vi "Start Async.vi"(8 "error in (no error)":errorcluster, 11 "OOP Server in":refnum<class "Template Server.lvclass">) -> (0 "error out":errorcluster, 3 "OOP Server out":refnum<class "Template Server.lvclass">)   [LabVIEW 2019, in "Template Server.lvlib" / "Template Server.lvclass"]
uses:
  Template Server.lvclass
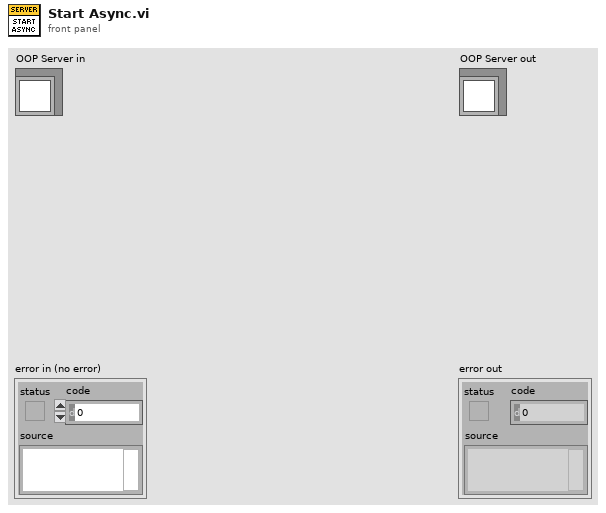
[diagram p1: front panel]
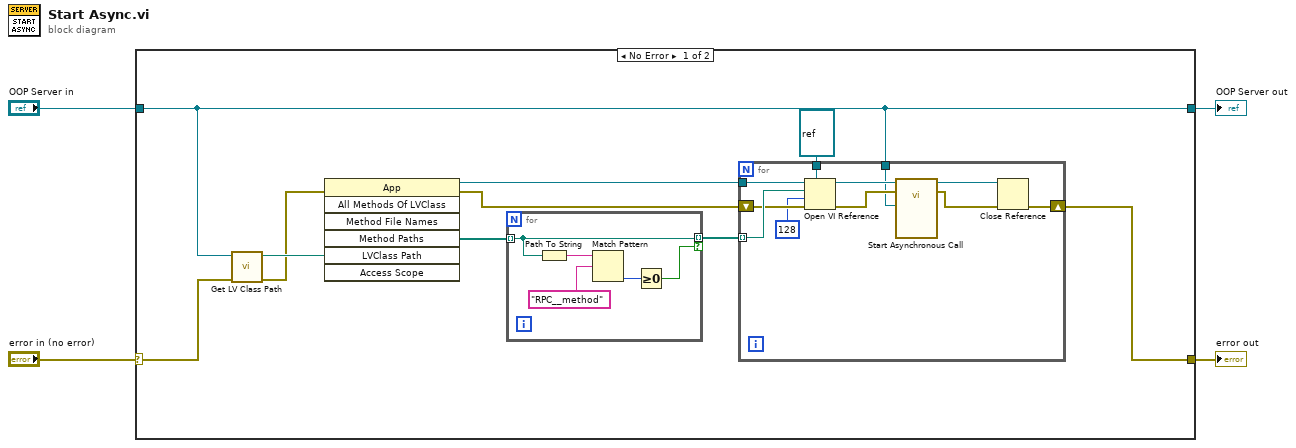
[diagram p0: block diagram]
diagram:
  n1 = case shown="No Error" "error in (no error)" {
    selector: "error in (no error)" -> [w8 w32]
    tunnel: [w5 w32] -> w3
    tunnel: [w9 w31] -> w1
    tunnel: "OOP Server in" -> [w9 w31]
    frame No Error {
      n2 = call <vilib>:"Get LV Class Path.vi"("error in (no error)"=w8, "object"=w9) -> ("error out"=w6:errorcluster, "class path"=w14:path)  [unwired: 8 in]
      n3 = invoke class="App" method="All Methods Of LVClass"(error in=w6, "LVClass Path"=w14) -> (reference out=w10:refnum<vi>, error out=w7:errorcluster, "Method Paths"=w13:path[])  [unwired: 5 in, 4 out]
      n4 = for {
        tunnel: w13 -> [w29] mode=indexing
        tunnel: [w29] -> w12 mode=indexing if=w26
        n5 = Path To String(path=w29) -> (string=w30:string)
        n6 = Match Pattern(string=w30, regular expression="RPC__method") -> (offset past match=w27:i32)  [unwired: 1 in, 3 out]
        n7 = Greater Or Equal To 0?(x=w27) -> (x >= 0?=w26:bool)
      }
      n8 = for {
        tunnel: w12 -> [w25] mode=indexing
        tunnel: refnum<vi> refnum ("type specifier VI Refnum (for type only)") -> [w24]
        tunnel: w10 -> [w21]
        tunnel: w9 -> [w18]
        shift-right: [w16] -> w5
        shift-left: w7 -> [w17]
        n9 = Open VI Reference(type specifier VI Refnum (for type only)=w24, application reference (local)=w21, vi path=w25, options=128 ("call and forget"), error in (no error)=w17) -> (vi reference=w23:refnum<vi>, error out=w20:errorcluster)  [unwired: 1 in]
        n10 = call-by-ref "Start Asynchronous Call"(reference=w23, error in=w20, "OOP Server in"=w18) -> (reference out=w22:refnum<vi>, error out=w19:errorcluster)  [unwired: 9 in, 2 out]
        n11 = Close Reference(reference=w22, error in (no error)=w19) -> (error out=w16:errorcluster)
      }
    }
    frame Error {
    }
  }
  "error out" <- w3
  "OOP Server out" <- w1
